vi "SSH_Read.vi"(8 "error in (no error)":errorcluster, 11 "Python":T1) -> (0 "error out":errorcluster, 2 "Reply":string, 3 "Python":T1)   [LabVIEW 2021]
uses:
  PythonCtrl.ctl
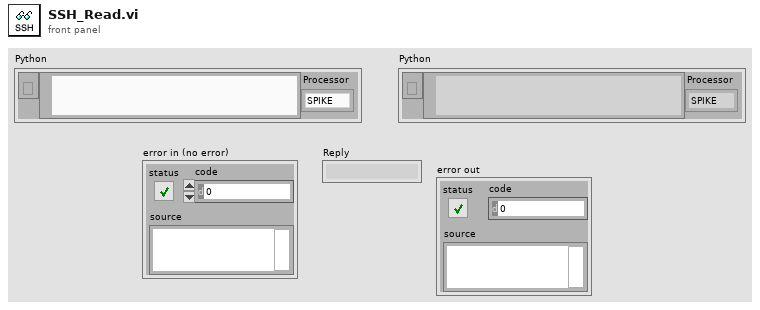
[diagram p1: front panel]
types:
  T1 = typedef "PythonCtrl.ctl" = cluster{"session":refnum<k35>, "PyPath":path, "Processor":enum16{"SPIKE", "Pi", "Pi_ssh"}}
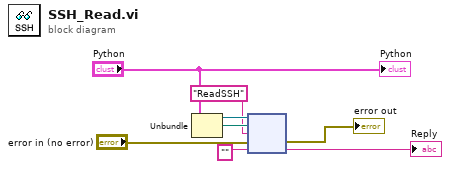
[diagram p0: block diagram]
diagram:
  n1 = Unbundle("Python") -> ("session"=w7:refnum<k35>, "PyPath"=w8:path)  [unwired: 1 out]
  n2 = node(w7, w8, "ReadSSH" ("function name"), "error in (no error)", "" ("replace string (\"\")")) -> (→"error out":errorcluster, →"Reply":string)  [unwired: 3 out]
  "Python" <- "Python"
